vi "Example.vi"() -> ()   [LabVIEW 2015]
uses:
  <vilib>/LV-Control-Refs/LV-Control-Refs.xnode
panel:
  in  "stop":bool
  out "Waveform Chart":dbl(graph)
  in  "Numeric Control":dbl
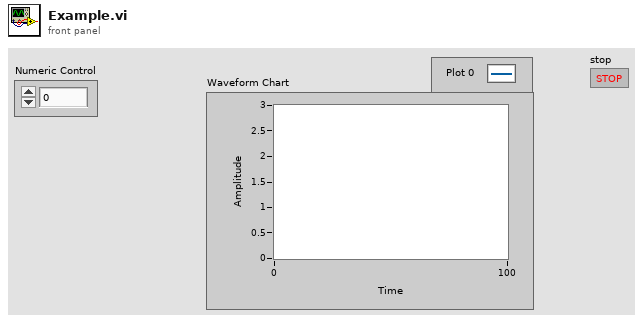
[diagram p1: front panel]
types:
  T1 = cluster{"Numeric Control":refnum<vi>, "Waveform Chart":refnum<vi>, "stop":refnum<vi>}
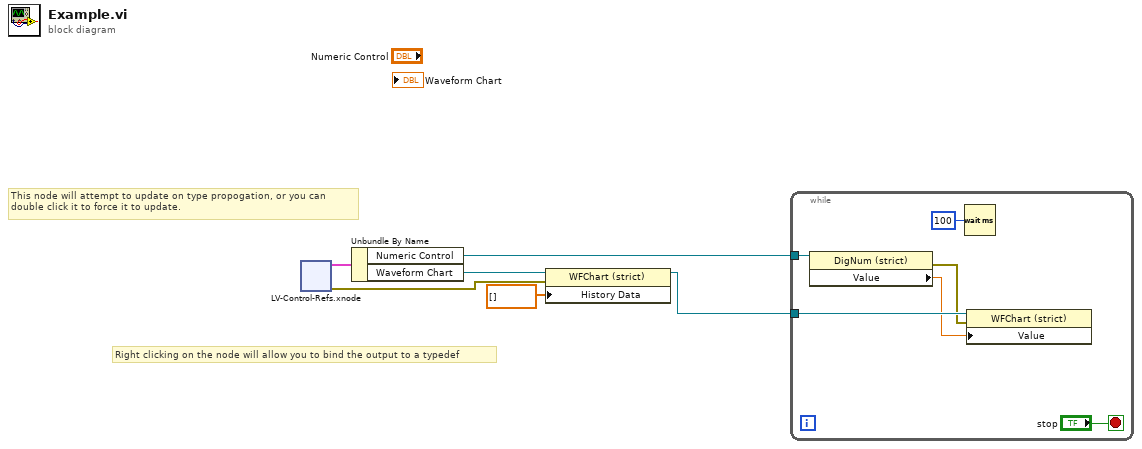
[diagram p0: block diagram]
diagram:
  # "Right clicking on the node will allow you to bind the output to a typedef"
  # "This node will attempt to update on type propogation, or you can\ndouble click it to force it to update."
  n1 = xnode "LV-Control-Refs.xnode"() -> ("Error Out"=w1:errorcluster, "Control Refs"=w2:T1)  [unwired: 1 in]
  n2 = Unbundle By Name(w2) -> ("Numeric Control"=w4:refnum<vi>, "Waveform Chart"=w5:refnum<vi>)
  n3 = property class="WFChart (strict)"(reference=w5, error in=w1, "History Data"=dbl[] []) -> (reference out=w3:refnum<vi>)  [unwired: 1 out]
  n4 = while {
    tunnel: w4 -> [w12]
    tunnel: w3 -> [w11]
    stop <- "stop" stop-if-true
    n5 = property class="DigNum (strict)"(reference=w12) -> (error out=w7:errorcluster, "Value"=w8:dbl)  [unwired: 1 in, 1 out]
    n6 = Wait (ms)(milliseconds to wait=u32 100) -> ()  [unwired: 1 out]
    n7 = property class="WFChart (strict)"(reference=w11, error in=w7, "Value"=w8) -> ()  [unwired: 2 out]
  }
